vi "oax_gsSelect File.vi"(4 "prompt":string, 5 "file names":string[](array[string])) -> (0 "canceled":bool, 1 "index":i32, 2 "file name":string)   [LabVIEW 2017]
panel:
  in  "Files":i32(listbox)
  in  "Cancel":bool
  in  "OK":bool
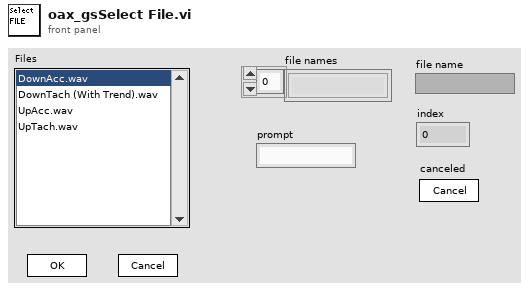
[diagram p1: front panel]
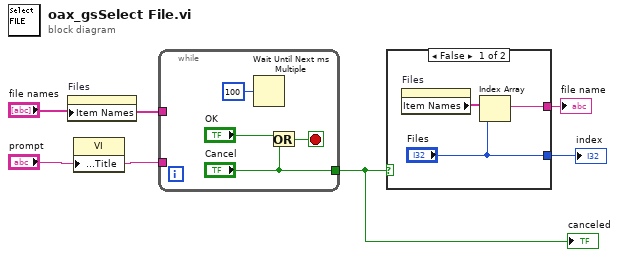
[diagram p0: block diagram]
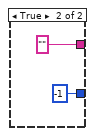
[diagram p2: hidden frame]
diagram:
  n1 = property on="Files" class="LstBox (strict)"("Item Names"="file names") -> ()  [unwired: 2 in, 2 out]
  n2 = property class="VI"("Front Panel Window:Title"="prompt") -> ()  [unwired: 2 in, 2 out]
  n3 = while {
    tunnel: ["Cancel"] -> w5
    tunnel: "file names" -> [_]
    tunnel: "prompt" -> [_]
    stop <- w8 stop-if-true
    n4 = Wait Until Next ms Multiple(millisecond multiple=u32 100) -> ()  [unwired: 1 out]
    n5 = Or(x="OK", y="Cancel") -> (x .or. y?=w8:bool)
  }
  "canceled" <- w5
  n6 = case shown="False" w5 {
    tunnel: [w11 ""] -> w4
    tunnel: ["Files" -1 ("Wave Files")] -> w3
    frame False {
      n7 = property on="Files" class="LstBox (strict)"() -> ("Item Names"=w12:string[])  [unwired: 2 in, 2 out]
      n8 = Index Array(array=w12, index="Files") -> (element=w11:string)
    }
    frame True {
    }
  }
  "file name" <- w4
  "index" <- w3
